vi "Region.vi"(11 "Test Case In":refnum<class "Test.Camera.lvclass">) -> (0 "error out":errorcluster, 3 "Test Case Out":refnum<class "Test.Camera.lvclass">)   [LabVIEW 2020, in "Test.Camera.lvclass"]
uses:
  Test.Camera.lvclass
  Test.Camera.lvclass/Test.Camera.ctl
  <vilib>/Astemes/LUnit/Test Case.lvclass
  c3e2611f-c54f-4219-a549-b8da21c7f085.vi
  0aa1576c-e916-4ad0-9a97-64bd3e4eb69b.vi
  g_industrial_cam/Camera/Camera.lvclass
  759e5037-5df0-4144-95b6-409846063909.vi
  g_industrial_cam/Camera/Image Offset.ctl
  C:/Program Files (x86)/National Instruments/LabVIEW 2020/vi.lib/Astemes/LUnit/Test Case.lvclass
  C:/Program Files (x86)/National Instruments/LabVIEW 2020/vi.lib/Astemes/LUnit/LUnit Runnable.lvclass
  C:/serenial/lib/g-industrial-camera/LabVIEW/tests/Test.Camera/Test.Camera.lvclass
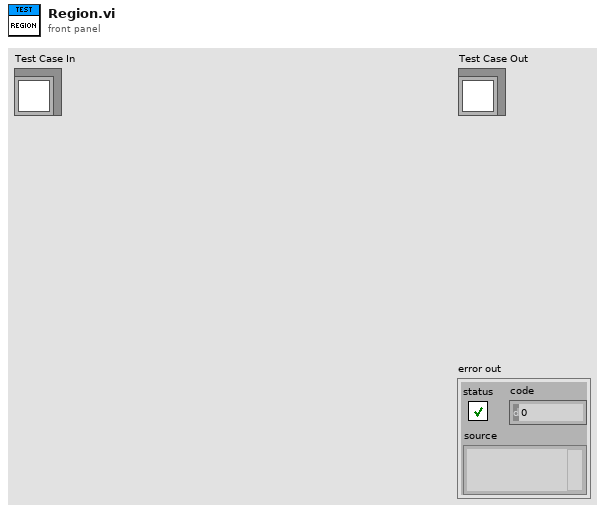
[diagram p1: front panel]
types:
  T1 = typedef "Camera.lvclass/Image Offset.ctl" = cluster{"x":i32, "y":i32}
  T2 = typedef "Buffer.lvclass/Image Size.ctl" = cluster{"Width":u16, "Height":u16}
  T3 = cluster{"Y Offset Increment":i32, "Y Offset Min":i32, "Y Offset Max":i32, "X Offset Increment":i32, "X Offset Min":i32, "X Offset Max":i32, "Offset Avaliable":bool, "Increment":i32, "Height Min":i32, "Height Max":i32, "Width Increment":i32, "Width Min":i32, "Width Max":i32, "Sensor Size":T2, "Region Offset":T1, "Region Size":T2}
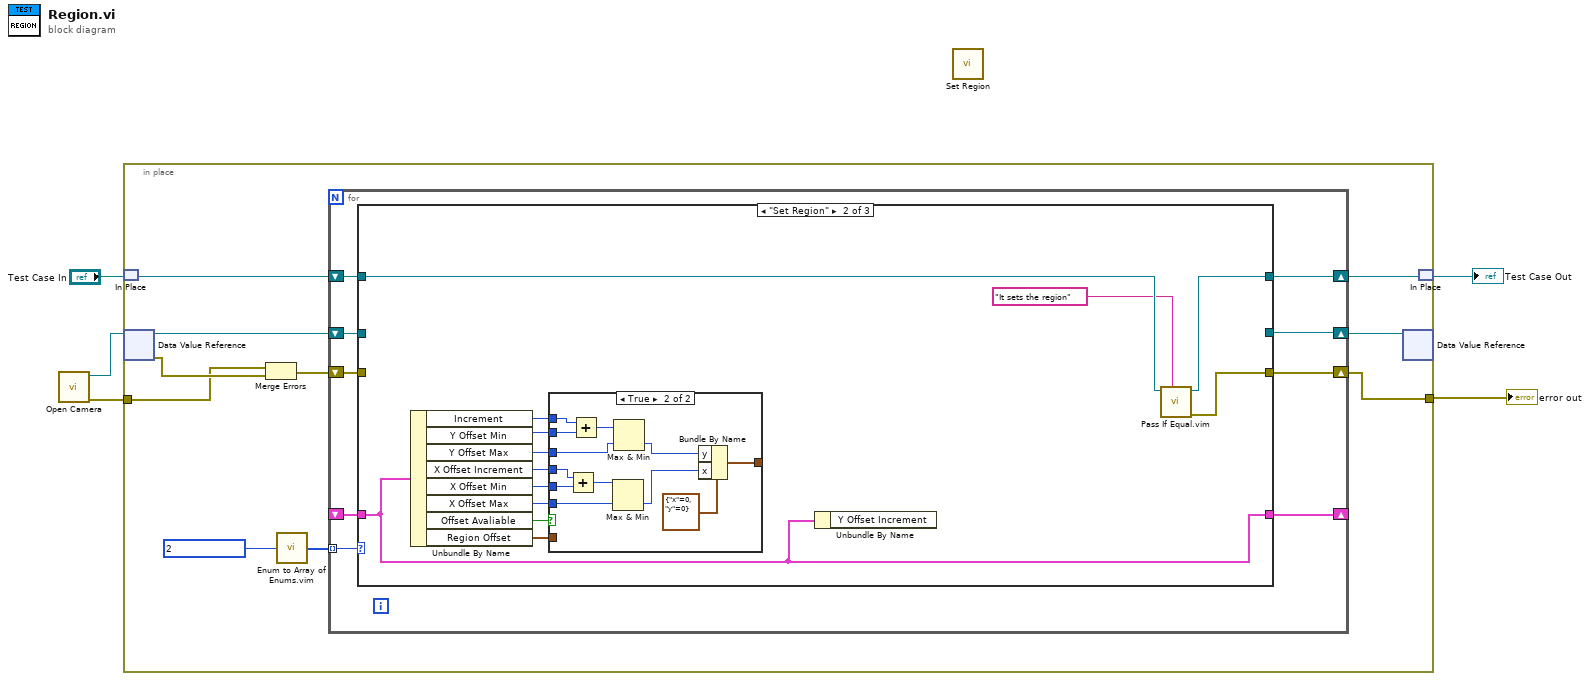
[diagram p0: block diagram]
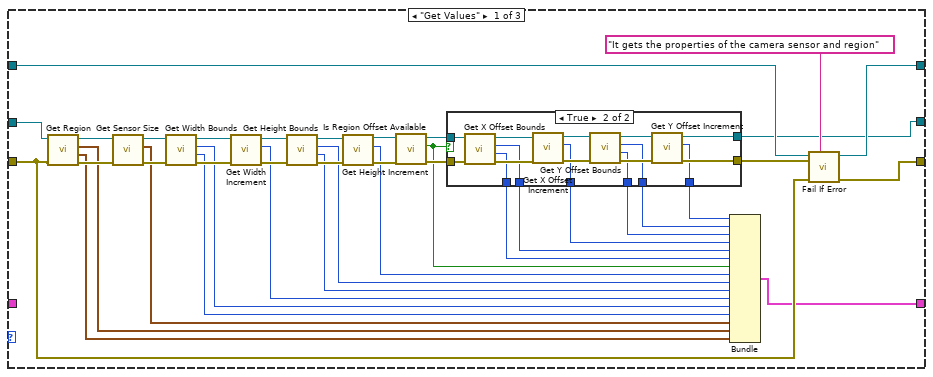
[diagram p2: hidden frame]
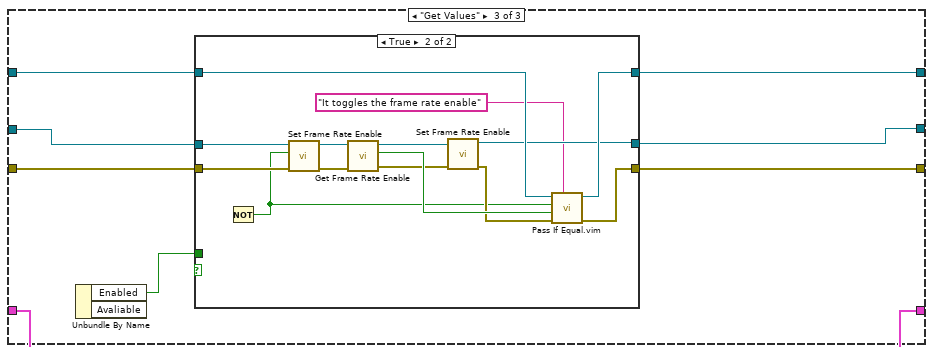
[diagram p5: hidden frame]
diagram:
  n1 = call "Open Camera.vi"() -> ("error out"=w5:errorcluster, "Camera"=w4:refnum<data-value>)  [unwired: 10 in]
  n2 = in-place {
    in-place-border: w5 -> [w8]
    in-place-border: [w7] -> w2
    n3 = in-place-match #1("Test Case In") -> (w10:refnum<class "Test.Camera.lvclass">)
    n4 = in-place-dvr #2(w4) -> (w14:refnum<class "Camera.lvclass">, w15:errorcluster)
    n5 = Merge Errors(w8, w15) -> (w13:errorcluster)
    n6 = call "Enum to Array of Enums.vim"("enum"=enum16{"Get Values", "Set Region"} 2) -> ("array of enums"=w11:enum16{"Get Values", "Set Region"}[])
    n7 = for {
      tunnel: w11 -> [w22] mode=indexing
      shift-right: [w21] -> w9
      shift-left: w14 -> [w24]
      shift-right: [w20] -> _
      shift-left: _ -> [w19]
      shift-right: [w17] -> w6
      shift-left: w10 -> [w18]
      shift-right: [w16] -> w7
      shift-left: w13 -> [w23]
      n8 = case shown="\"Set Region\"" w22 {
        tunnel: w24 -> [w57 _ w114]
        tunnel: w23 -> [w58 _ w115]
        tunnel: [w25 _ w110] -> w21
        tunnel: [w26 w82 w108] -> w20
        tunnel: w19 -> [_ w82 w108]
        tunnel: w18 -> [w62 w94 w112]
        tunnel: [w61 w93 w111] -> w17
        tunnel: [w59 w92 w109] -> w16
        frame "Get Values" {
          n9 = call "Get Region.vi"("error in (no error)"=w58, "Camera in"=w57) -> ("error out"=w63:errorcluster, "Region Size"=w56:T2, "Region Offset"=w55:T1, "Camera"=w54:refnum<class "Camera.lvclass">)  [unwired: 6 in]
          n10 = call "Get Sensor Size.vi"("error in (no error)"=w63, "Camera in"=w54) -> ("error out"=w51:errorcluster, "Sensor Size"=w45:T2, "Camera"=w53:refnum<class "Camera.lvclass">)  [unwired: 7 in]
          n11 = call "Get Width Bounds.vi"("error in (no error)"=w51, "Camera in"=w53) -> ("error out"=w50:errorcluster, "Width Max"=w44:i32, "Width Min"=w43:i32, "Camera"=w52:refnum<class "Camera.lvclass">)  [unwired: 6 in]
          n12 = call "Get Width Increment.vi"("error in (no error)"=w50, "Camera in"=w52) -> ("error out"=w49:errorcluster, "Width Increment"=w42:i32, "Camera"=w48:refnum<class "Camera.lvclass">)  [unwired: 7 in]
          n13 = call "Get Height Bounds.vi"("error in (no error)"=w49, "Camera in"=w48) -> ("error out"=w47:errorcluster, "Height Max"=w41:i32, "Height Min"=w40:i32, "Camera"=w46:refnum<class "Camera.lvclass">)  [unwired: 6 in]
          n14 = call "Get Height Increment.vi"("error in (no error)"=w47, "Camera in"=w46) -> ("error out"=w39:errorcluster, "Increment"=w37:i32, "Camera"=w38:refnum<class "Camera.lvclass">)  [unwired: 7 in]
          n15 = call "Is Region Offset Available.vi"("error in (no error)"=w39, "Camera in"=w38) -> ("error out"=w36:errorcluster, "Offset Avaliable"=w27:bool, "Camera"=w35:refnum<class "Camera.lvclass">)  [unwired: 7 in]
          n16 = case shown="True" w27 {
            tunnel: w36 -> [w65 w81]
            tunnel: w35 -> [w64 w80]
            tunnel: [_ w73] -> w34
            tunnel: [_ w72] -> w33
            tunnel: [_ w71] -> w32
            tunnel: [_ w70] -> w31
            tunnel: [_ w69] -> w30
            tunnel: [w65 w68] -> w29
            tunnel: [_ w67] -> w28
            tunnel: [w64 w66] -> w25
            frame False {
            }
            frame True {
              n17 = call "Get X Offset Bounds.vi"("error in (no error)"=w81, "Camera in"=w80) -> ("error out"=w79:errorcluster, "X Offset Max"=w73:i32, "X Offset Min"=w72:i32, "Camera"=w76:refnum<class "Camera.lvclass">)  [unwired: 6 in]
              n18 = call "Get X Offset Increment.vi"("error in (no error)"=w79, "Camera in"=w76) -> ("error out"=w78:errorcluster, "X Offset Increment"=w71:i32, "Camera"=w75:refnum<class "Camera.lvclass">)  [unwired: 7 in]
              n19 = call "Get Y Offset Bounds.vi"("error in (no error)"=w78, "Camera in"=w75) -> ("error out"=w77:errorcluster, "Y Offset Max"=w70:i32, "Y Offset Min"=w69:i32, "Camera"=w74:refnum<class "Camera.lvclass">)  [unwired: 6 in]
              n20 = call "Get Y Offset Increment.vi"("error in (no error)"=w77, "Camera in"=w74) -> ("error out"=w68:errorcluster, "Y Offset Increment"=w67:i32, "Camera"=w66:refnum<class "Camera.lvclass">)  [unwired: 7 in]
            }
          }
          n21 = Bundle("Y Offset Increment"=w28, "Y Offset Min"=w30, "Y Offset Max"=w31, "X Offset Increment"=w32, "X Offset Min"=w33, "X Offset Max"=w34, "Offset Avaliable"=w27, "Increment"=w37, "Height Min"=w40, "Height Max"=w41, "Width Increment"=w42, "Width Min"=w43, "Width Max"=w44, "Sensor Size"=w45, "Region Offset"=w55, "Region Size"=w56) -> (w26:T3)  [unwired: 1 in]
          n22 = call <vilib>:"Fail If Error.vi"("Description"="It gets the properties of the camera sensor and region", "error in (no error)"=w58, "Assert error"=w29, "LUnit Test Case In"=w62) -> ("error out"=w59:errorcluster, "LUnit Test Case Out"=w61:refnum<class "Test.Camera.lvclass">)  [unwired: 6 in]
        }
        frame "Set Region" {
          n23 = Unbundle By Name(w82) -> ("Increment"=w88:i32, "Y Offset Min"=w89:i32, "Y Offset Max"=w85:i32, "X Offset Increment"=w86:i32, "X Offset Min"=w87:i32, "X Offset Max"=w84:i32, "Offset Avaliable"=w90:bool, "Region Offset"=w83:T1)
          n24 = case shown="True" w90 {
            tunnel: [w95 w96] -> _
            tunnel: w89 -> [_ w107]
            tunnel: w88 -> [_ w106]
            tunnel: w87 -> [_ w105]
            tunnel: w86 -> [_ w104]
            tunnel: w85 -> [_ w102]
            tunnel: w84 -> [_ w100]
            tunnel: w83 -> [w95 _]
            frame False {
            }
            frame True {
              n25 = Add(x=w104, y=w105) -> (x+y=w101:i32)
              n26 = Add(x=w106, y=w107) -> (x+y=w103:i32)
              n27 = Max & Min(x=w101, y=w100) -> (min(x,y)=w99:i32)  [unwired: 1 out]
              n28 = Max & Min(x=w103, y=w102) -> (min(x,y)=w98:i32)  [unwired: 1 out]
              n29 = Bundle By Name(cluster=T1 {"x"=0, "y"=0} ("Image Offset"), "y"=w98, "x"=w99) -> (w96:T1)
            }
          }
          n30 = Unbundle By Name(w82) -> ()  [unwired: 1 out]
          n31 = call "Pass If Equal.vim"("Description"="It sets the region", "LUnit Test Case In"=w94) -> ("error out"=w92:errorcluster, "LUnit Test Case Out"=w93:refnum<class "Test.Camera.lvclass">)  [unwired: 8 in]
        }
        frame "Get Values" {
          n32 = Unbundle By Name() -> ("Enabled"=w113:bool)  [unwired: 1 in, 1 out]
          n33 = case shown="True" {
            selector: _ -> [_ _]
            tunnel: w115 -> [w118 w129]
            tunnel: w114 -> [w117 w128]
            tunnel: w113 -> [_ _]
            tunnel: w112 -> [w116 w130]
            tunnel: [w116 w131] -> w111
            tunnel: [w117 w121] -> w110
            tunnel: [w118 w132] -> w109
            frame False {
            }
            frame True {
              n34 = Not() -> (.not. x?=w119:bool)  [unwired: 1 in]
              n35 = call "Set Frame Rate Enable.vi"("error in (no error)"=w129, "Enable"=w119, "Camera in"=w128) -> ("error out"=w127:errorcluster, "Camera"=w126:refnum<class "Camera.lvclass">)  [unwired: 7 in]
              n36 = call "Get Frame Rate Enable.vi"("error in (no error)"=w127, "Camera in"=w126) -> ("error out"=w124:errorcluster, "Enabled"=w125:bool, "Camera"=w123:refnum<class "Camera.lvclass">)  [unwired: 7 in]
              n37 = call "Set Frame Rate Enable.vi"("error in (no error)"=w124, "Camera in"=w123) -> ("error out"=w122:errorcluster, "Camera"=w121:refnum<class "Camera.lvclass">)  [unwired: 8 in]
              n38 = call "Pass If Equal.vim"("Description"="It toggles the frame rate enable", "error in (no error)"=w122, "Actual"=w125, "Expected"=w119, "LUnit Test Case In"=w130) -> ("error out"=w132:errorcluster, "LUnit Test Case Out"=w131:refnum<class "Test.Camera.lvclass">)  [unwired: 5 in]
            }
          }
        }
      }
    }
    n39 = in-place-dvr #2(w9) -> ()  [unwired: 2 out]
    n40 = in-place-match #1(w6) -> (→"Test Case Out":refnum<class "Test.Camera.lvclass">)
  }
  "error out" <- w2
  n41 = call "Set Region.vi"() -> ()  [unwired: 10 in, 2 out]
